vi "Tank2 GO!.vi"() -> ()   [LabVIEW 2012]
doc: "This VI demonstrates how to control a simulated Robotics Starter Kit 2.0 robot. With a few modifications, you can deploy this VI to the Single-Board RIO 9632 on a real robot, and it runs on the real-time controller. For more information about how to modify this VI so you can deploy it to real hardware, refer to the <B>Robotics Module>>Simulating Mobile Robots</B> book on the <B>Contents</B> tab of the LabVIEW Help."
uses:
  <vilib>/Platform/TimedLoop/XDataNode/timing_clust.ctl
  <vilib>/Platform/TimedLoop/XDataNode/nitl_modes.ctl
  <vilib>/Platform/TimedLoop/XDataNode/wakeup.ctl
  <vilib>/robotics/Starter Kit/2.0/9632 Host Interface/NI_Robotics_Starter Kit Host_9632_2.0.lvclass
  <vilib>/Utility/AngleManip/Degrees to Radians (Scalar DBL).vi
  <vilib>/robotics/Steering/Steering Frame/Apply Steering Frame Velocity to Motors.vi
  <vilib>/Platform/TimedLoop/XDataNode/XDataNode.xnode
  <vilib>/Platform/TimedLoop/XDataNode/XDNodeRunTimeDep.lvlib
  <vilib>/Utility/AngleManip/NI_AngleManipulation.lvlib
  <vilib>/robotics/Utilities/Scan Angles/NI_Robotics_Scan Angles.lvlib
  <vilib>/robotics/Steering/Steering Frame/NI_Robotics_Steering Frame.lvclass
  <vilib>/robotics/Starter Kit/Host Interface/NI_Robotics_Starter Kit Host.lvclass
  <vilib>/robotics/Starter Kit/2.0/NI_Robotics_Starter Kit Host_2.0.lvlib
panel:
  out "Sensor Data":cluster{"angles (deg)":dbl[], "distances":dbl[]}(graph)
  in  "stop":bool
  # "This VI demonstrates how to control a simulated Robotics Starter Kit 2.0 robot.\n\nRun this VI to launch the simulation.  The simulated environment is displayed in a separate window.  The graph displays the range data acquired by the simulated ultrasonic sensor on the robot.  Click the STOP button to end the simulation."
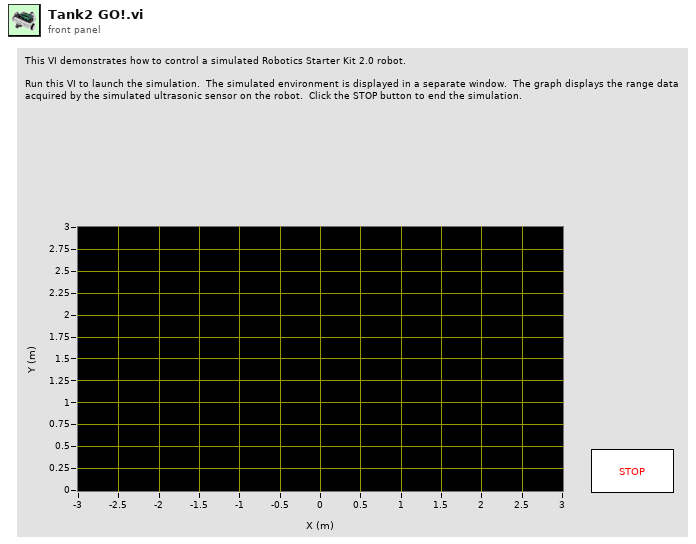
[diagram p1: front panel]
types:
  T1 = typedef "NI_Robotics_Scan Angles.lvlib/Scan Angle Data.ctl" = cluster{"angles":dbl[], "distances":dbl[], "current index":i32, "previous index":i32}
  T2 = typedef "XDNodeRunTimeDep.lvlib/timing_clust.ctl" = cluster{"Expected End [f-1]":u64, "Actual End [f-1]":u64, "Finished Late? [f-1]":bool, "Expected End [i-1]":u64, "Actual End [i-1]":u64, "Finished Late? [i-1]":bool, "Expected Start [i]":u64, "Actual Start [i]":u64, "Expected Start [f]":u64, "Actual Start [f]":u64, "Source Name":string, "Structure Name":string, "Period":i64, "Deadline":i64, "Offset":i64, "Start":i64, "Priority":i32, "Timeout":i32, "Mode":T3, "Wakeup Reason":T4, "Error":errorcluster, "Source Type":string, "Secondary Source Type":string, "Global End Time":u64, "Global Start Time":u64, "Frame Duration":u64, "Iteration Duration":u64, "Assigned CPU":i32, "I/O Scan Engine Mode":u32}
  T3 = typedef "XDNodeRunTimeDep.lvlib/nitl_modes.ctl" = enum32{"No Change", "Process missed periods, maintain original phase", "Discard missed periods, maintain original phase", "Process missed periods, ignore original phase", "Discard missed periods, ignore original phase"}
  T4 = typedef "XDNodeRunTimeDep.lvlib/wakeup.ctl" = enum32{"Normal", "Aborted", "Asynchronous wakeup", "Timing source error", "Timed loop error", "Timeout"}
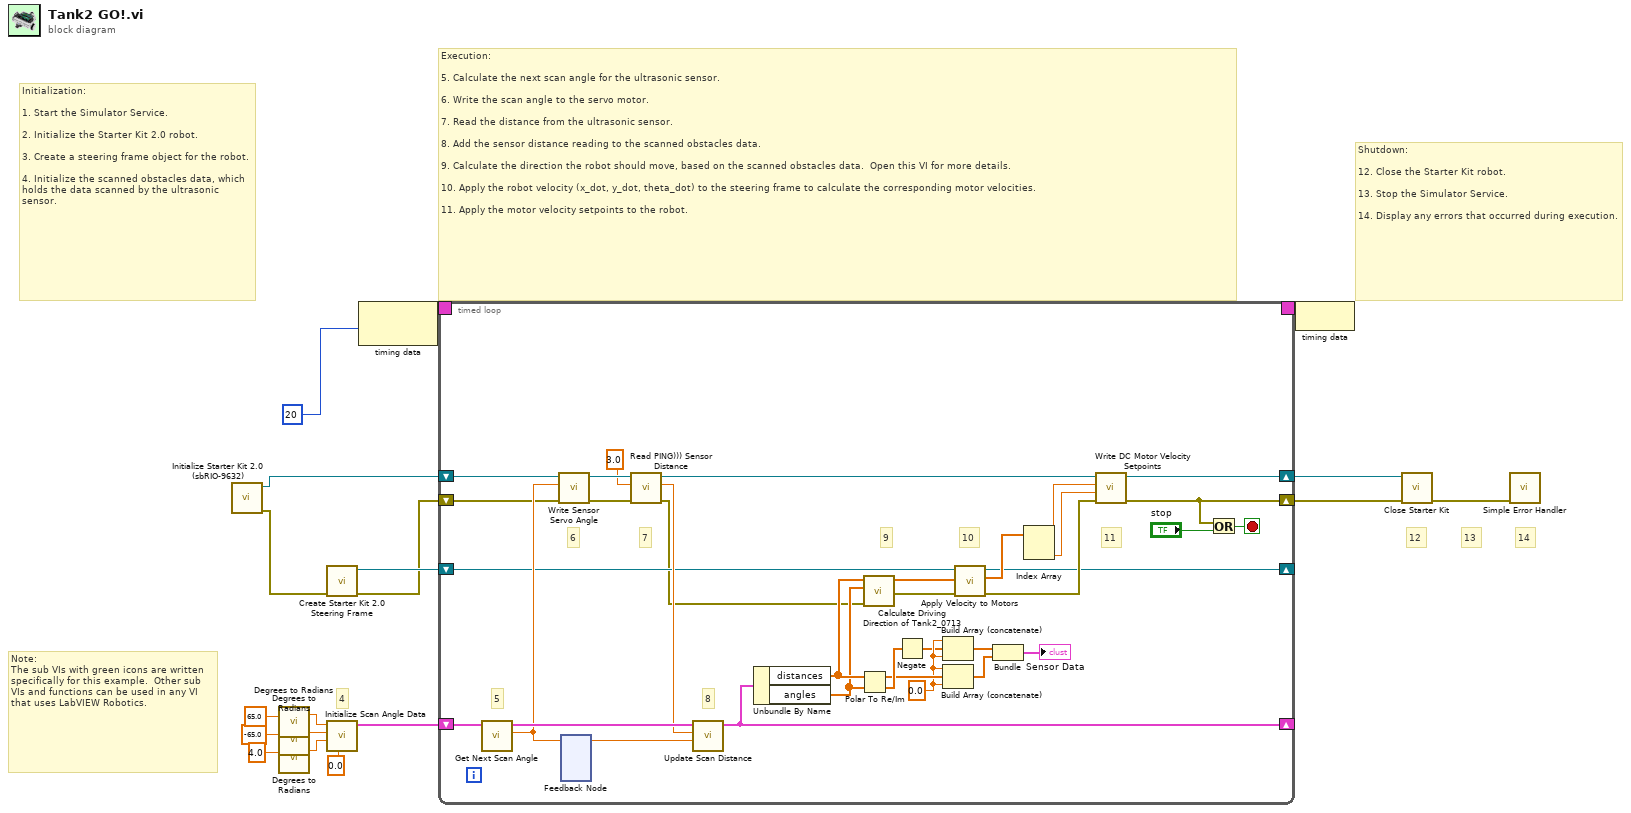
[diagram p0: block diagram]
diagram:
  # "14"
  # "13"
  # "12"
  # "Execution:\n\n5. Calculate the next scan angle for the ultrasonic sensor.\n\n6. Write the scan angle to the servo motor.\n\n7. Read the distance from the ultrasonic sensor.\n\n8. Add the sensor distance reading to the scanned obstacles data.\n\n9. Calculate the direction the robot should move, based on the scanned obstacles data.  Open this VI for more details.\n\n10. Apply the robot velocity (x_dot, y_dot, theta_dot) to the steering frame to calculate the corresponding motor velocities.\n\n11. Apply the motor velocity setpoints to the robot."
  # "Shutdown:\n\n12. Close the Starter Kit robot.\n\n13. Stop the Simulator Service.\n\n14. Display any errors that occurred during execution."
  # "Note:\nThe sub VIs with green icons are written specifically for this example.  Other sub VIs and functions can be used in any VI that uses LabVIEW Robotics."
  # "4"
  # "Initialization:\n\n1. Start the Simulator Service.\n\n2. Initialize the Starter Kit 2.0 robot.\n\n3. Create a steering frame object for the robot.\n\n4. Initialize the scanned obstacles data, which holds the data scanned by the ultrasonic sensor."
  n1 = call <vilib>:"Initialize Starter Kit 2.0 (sbRIO-9632).vi"() -> ("error out"=w2:errorcluster, "FPGA starter kit host 2.0 out"=w3:refnum<class "NI_Robotics_Starter Kit Host_9632_2.0.lvclass">)  [unwired: 10 in]
  n2 = call-poly <vilib>:"Degrees to Radians.vi"("angle (deg)"=65.0 ("max angle")) -> ("angle (rad)"=w11:dbl)  [unwired: 2 in]
  n3 = call-poly <vilib>:"Degrees to Radians.vi"("angle (deg)"=-65.0 ("min angle")) -> ("angle (rad)"=w7:dbl)  [unwired: 2 in]
  n4 = call-poly <vilib>:"Degrees to Radians.vi"("angle (deg)"=4.0 ("scan angle")) -> ("angle (rad)"=w8:dbl)  [unwired: 2 in]
  n5 = call <vilib>:"Create Starter Kit 2.0 Steering Frame.vi"("error in (no error)"=w2) -> ("error out"=w5:errorcluster, "starter kit differential steering frame"=w15:refnum<class "NI_Robotics_Differential Steering Frame.lvclass">)  [unwired: 9 in]
  n6 = call <vilib>:"Initialize Scan Angle Data.vi"("initial angle (0)"=0.0, "scan angle"=w8, "min angle"=w7, "max angle"=w11) -> ("scan angles"=w6:T1)  [unwired: 6 in, 1 out]
  n7 = node-c288(i64 20 ("Period")) -> (w18:T2)
  n8 = timed-loop {
    shift-right: [w33] -> w14
    shift-left: w3 -> [w38]
    shift-right: [w22] -> w13
    shift-left: w5 -> [w35]
    shift-right: [w36] -> _
    shift-left: w15 -> [w37]
    timing: w18 -> [_]
    timing-out: [_] -> w17
    shift-right: [w32] -> _
    shift-left: w6 -> [w39]
    stop <- w34 stop-if-true
    w28 = 0.0 ("element")
    # "7"
    # "6"
    # "11"
    # "10"
    # "9"
    # "8"
    # "5"
    n9 = call <vilib>:"Get Next Scan Angle.vi"("scan angles in"=w39) -> ("new angle"=w48:dbl, "scan angles out"=w51:T1)  [unwired: 9 in]
    n10 = call <vilib>:"Write Sensor Servo Angle.vi"("error in (no error)"=w35, "ccw servo angle (rad)"=w48, "starter kit host in"=w38) -> ("error out"=w45:errorcluster, "starter kit host out"=w46:refnum<class "NI_Robotics_Starter Kit Host_9632_2.0.lvclass">)  [unwired: 7 in]
    n11 = feedback #1() -> (w50:dbl)  [unwired: 1 in]
    n12 = feedback-in #1(w48) -> ()
    n13 = call <vilib>:"Read PING))) Sensor Distance.vi"("error in (no error)"=w45, "default distance (NaN)"=3.0, "starter kit host in"=w46) -> ("error out"=w21:errorcluster, "distance (m)"=w47:dbl, "starter kit host out"=w44:refnum<class "NI_Robotics_Starter Kit Host_9632_2.0.lvclass">)  [unwired: 5 in, 1 out]
    n14 = call <vilib>:"Update Scan Distance.vi"("scan angle"=w50, "new scan distance"=w47, "scan angles in"=w51) -> ("scan angles out"=w32:T1)  [unwired: 8 in]
    n15 = Unbundle By Name(w32) -> ("distances"=w24:dbl[], "angles"=w23:dbl[])
    n16 = Polar To Re/Im(2:w23, 3:w24) -> (0:w31:dbl[], 1:w30:dbl[])
    n17 = call "Calculate Driving Direction of Tank2_0713.vi"("error in (no error)"=w21, "obstacle angles (rad)"=w23, "obstacle distances (m)"=w24) -> ("error out"=w20:errorcluster, "steering frame velocity"=w19:dbl[])  [unwired: 7 in]
    n18 = Negate(x=w31) -> (-x=w26:dbl[])
    n19 = Build Array (concatenate)(w28, w26, w28) -> (w27:dbl[])
    n20 = Build Array (concatenate)(w28, w30, w28) -> (w29:dbl[])
    n21 = call-poly <vilib>:"Apply Velocity to Motors.vi"("error in (no error)"=w20, "steering frame velocity"=w19, "steering frame in"=w37) -> ("error out"=w43:errorcluster, "ccw motor velocity setpoints"=w49:dbl[], "steering frame out"=w36:refnum<class "NI_Robotics_Differential Steering Frame.lvclass">)  [unwired: 4 in, 2 out]
    n22 = Bundle(w27, w29) -> (→"Sensor Data":cluster{dbl[], dbl[]})  [unwired: 1 in]
    n23 = Index Array(array=w49) -> (element #1=w42:dbl, element #2=w41:dbl)  [unwired: 2 in]
    n24 = call <vilib>:"Write DC Motor Velocity Setpoints.vi"("error in (no error)"=w43, "right motor ccw velocity (rad/s)"=w41, "left motor ccw velocity (rad/s)"=w42, "starter kit host in"=w44) -> ("error out"=w22:errorcluster, "starter kit host out"=w33:refnum<class "NI_Robotics_Starter Kit Host_9632_2.0.lvclass">)  [unwired: 6 in]
    n25 = Or(x=w22, y="stop") -> (x .or. y?=w34:bool)
  }
  n26 = node-c288(w17) -> ()
  n27 = call-dynamic "Close Starter Kit.vi"("error in (no error)"=w13, "starter kit host in"=w14) -> ("error out"=w1:errorcluster)  [unwired: 9 in]
  n28 = call <vilib>:"Simple Error Handler.vi"("error in (no error)"=w1) -> ()  [unwired: 4 in, 5 out]
